vi "Shooter PID.vi"() -> ()   [LabVIEW 2020]
panel:
  in  "Shooter PID Constants":T1={"P Gain"=0.0, "I Gain"=0.0, "D Gain"=0.0, "F Gain"=0.0002195, "I Zone"=0.0, "Min Output"=-1.0, "Max Output"=1.0} {"Max Output" min=-1.0 max=1.0 step=0.01; "Min Output" min=-1.0 max=1.0 step=0.01; "I Zone" step=0.01; "F Gain" step=0.01; "D Gain" step=0.01; "I Gain" step=0.01; "P Gain" min=0.0 step=0.01}
  in  "Accelerator PID Constants":T1={"P Gain"=2e-05, "I Gain"=2e-08, "D Gain"=0.0, "F Gain"=0.000289, "I Zone"=0.0, "Min Output"=-1.0, "Max Output"=1.0} {"Max Output" min=-1.0 max=1.0 step=0.01; "Min Output" min=-1.0 max=1.0 step=0.01; "I Zone" step=0.01; "F Gain" step=0.01; "D Gain" step=0.01; "I Gain" step=0.01; "P Gain" min=inf step=0.01}
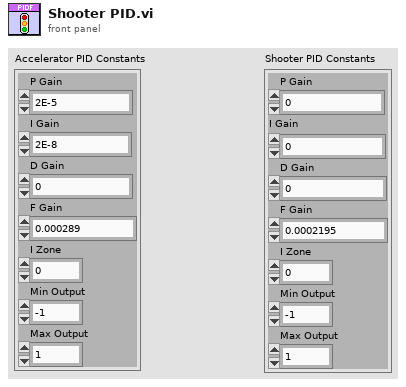
[diagram p1: front panel]
types:
  T1 = cluster{"P Gain":dbl, "I Gain":dbl, "D Gain":dbl, "F Gain":dbl, "I Zone":dbl, "Min Output":dbl, "Max Output":dbl}
  T2 = typedef "WPI_MotorControlDeviceRef.ctl" = cluster{"DeviceStatus":errorcluster, "Type":T3, "PWM":cluster{"PWM Channel":T4, "DeadBand":T5}, "CAN":cluster{"Device Number":u8, "SetOutput VI Ref":variant, "GetOutput VI Ref":variant, "Enable VI Ref":variant, "Disable VI Ref":variant, "Data":variant}, "Invert":bool, "DIO PWM":cluster{"PWM \"Enable\" Channel":T4, "DIOChannel":T6, "PWM Rate":dbl}}
  T3 = typedef "WPI_MotorControlType.ctl" = enum16{"PWM", "CAN", "DIO PWM"}
  T4 = typedef "FPGA_DIOPWMChannel.ctl" = enum8{"PWM 0", "PWM 1", "PWM 2", "PWM 3", "PWM 4", "PWM 5", "PWM 6", "PWM 7", "PWM 8", "PWM 9", "PWM MXP 0", "PWM MXP 1", "PWM MXP 2", "PWM MXP 3", "PWM MXP 4", "PWM MXP 5", "PWM MXP 6", "PWM MXP 7", "PWM MXP 8", "PWM MXP 9", "Invalid"}
  T5 = typedef "WPI_PWMDeadband.ctl" = cluster{"Name":string, "maxPositivePwm":i32, "minPositivePwm":i32, "centerPwm":i32, "maxNegativePwm":i32, "minNegativePwm":i32, "angularRange":u16}
  T6 = typedef "FPGA_DIOChannel.ctl" = enum8{"DIO 0", "DIO 1", "DIO 2", "DIO 3", "DIO 4", "DIO 5", "DIO 6", "DIO 7", "DIO 8", "DIO 9", "DIO MXP 0", "DIO MXP 1", "DIO MXP 2", "DIO MXP 3", "DIO MXP 4", "DIO MXP 5", "DIO MXP 6", "DIO MXP 7", "DIO MXP 8", "DIO MXP 9", "DIO MXP 10", "DIO MXP 11", "DIO MXP 12", "DIO MXP 13", "DIO MXP 14", "DIO MXP 15", "SPI Port CS1", "SPI Port CS2", "SPI Port CS3", "SPI Port MISO", "SPI Port MOSI", "Invalid"}
  T7 = cluster{"MotorControlDevRef":T2, "MotorControlDevRef":T2}
  T8 = cluster{"P Gain":bool, "I Gain":bool, "D Gain":bool, "F Gain":bool, "I Zone":bool, "Min Output":bool, "Max Output":bool}
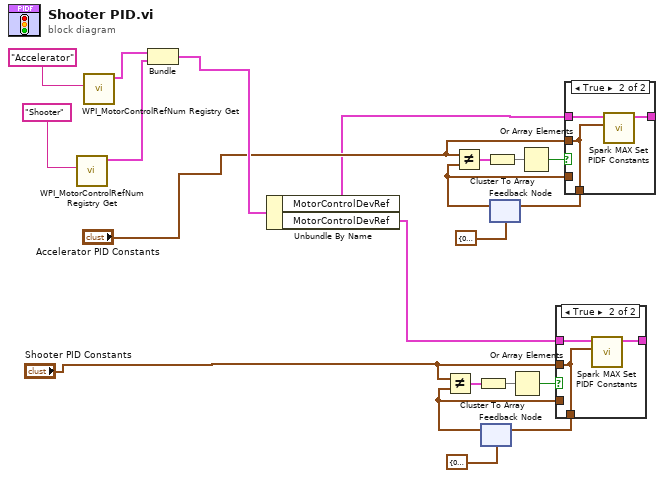
[diagram p0: block diagram]
diagram:
  n1 = call <vilib>:"WPI_MotorControlRefNum Registry Get.vi"("refnum name"="Shooter") -> ("MotorControlDevRef"=w18:T2)  [unwired: 9 in, 1 out]
  n2 = call <vilib>:"WPI_MotorControlRefNum Registry Get.vi"("refnum name"="Accelerator") -> ("MotorControlDevRef"=w19:T2)  [unwired: 9 in, 1 out]
  n3 = Bundle("MotorControlDevRef"=w19, "MotorControlDevRef"=w18) -> (w17:T7)  [unwired: 1 in]
  n4 = Unbundle By Name(w17) -> ("MotorControlDevRef"=w2:T2, "MotorControlDevRef"=w1:T2)
  n5 = feedback #1(T1 {"P Gain"=0.0, "I Gain"=0.0, "D Gain"=0.0, "F Gain"=0.0, "I Zone"=0.0, "Min Output"=0.0, "Max Output"=0.0} ("PID Constants")) -> (w14:T1)
  n6 = Not Equal?(x="Shooter PID Constants", y=w14) -> (x != y?=w9:T8)
  n7 = Cluster To Array(cluster=w9) -> (array=w10:bool[])
  n8 = feedback #2(T1 {"P Gain"=0.0, "I Gain"=0.0, "D Gain"=0.0, "F Gain"=0.0, "I Zone"=0.0, "Min Output"=0.0, "Max Output"=0.0} ("PID Constants")) -> (w8:T1)
  n9 = Not Equal?(x="Accelerator PID Constants", y=w8) -> (x != y?=w3:T8)
  n10 = Cluster To Array(cluster=w3) -> (array=w4:bool[])
  n11 = Or Array Elements(Boolean array=w10) -> (logical OR=w12:bool)
  n12 = Or Array Elements(Boolean array=w4) -> (logical OR=w6:bool)
  n13 = case shown="True" w12 {
    tunnel: w1 -> [w22 w26]
    tunnel: "Shooter PID Constants" -> [_ w24]
    tunnel: [w23 w24] -> w13
    tunnel: w14 -> [w23 _]
    tunnel: [w22 w25] -> _
    frame False {
    }
    frame True {
      n14 = call <vilib>:"Spark MAX Set PIDF Constants.vi"("PID Constants"=w24, "MotorControlDeviceRef"=w26) -> ("MotorControlDeviceRef"=w25:T2)  [unwired: 8 in, 1 out]
    }
  }
  n15 = feedback-in #1(w13) -> ()
  n16 = case shown="True" w6 {
    tunnel: w2 -> [w27 w29]
    tunnel: "Accelerator PID Constants" -> [_ w30]
    tunnel: [w28 w30] -> w7
    tunnel: w8 -> [w28 _]
    tunnel: [w27 w31] -> _
    frame False {
    }
    frame True {
      n17 = call <vilib>:"Spark MAX Set PIDF Constants.vi"("PID Constants"=w30, "MotorControlDeviceRef"=w29) -> ("MotorControlDeviceRef"=w31:T2)  [unwired: 8 in, 1 out]
    }
  }
  n18 = feedback-in #2(w7) -> ()
